vi "SPL Calc 2.0.vi"(9 "Gain":dbl(slide) min=0.0 max=50.0 scale=0.0..50.0, 10 "Voltage RMS Reference (V RMS/Pa)":dbl, 11 "Dynamic Data":dynamicdata(waveform)) -> (3 "SPL":dbl)   [LabVIEW 2020]
uses:
  <vilib>/measure/madcrms.llb/Basic Averaged DC-RMS for 1 Chan.vi
  <vilib>/measure/NI_MAPro.lvlib
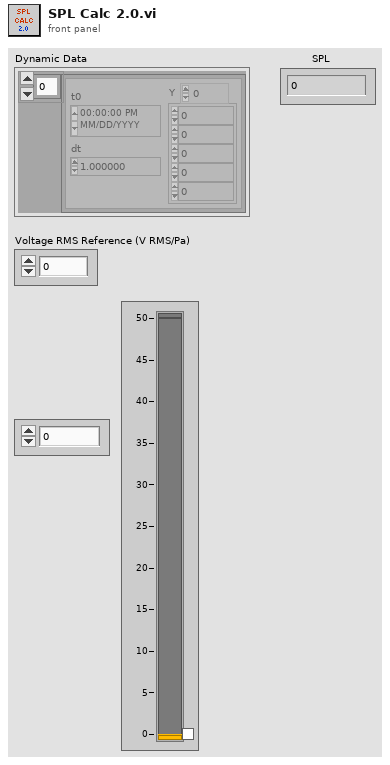
[diagram p1: front panel]
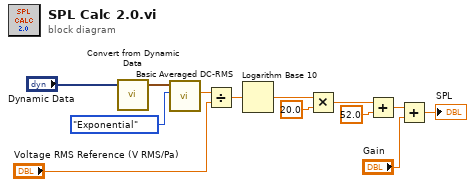
[diagram p0: block diagram]
diagram:
  n1 = call "Convert from Dynamic Data"("Dynamic Data Type"="Dynamic Data") -> ("Waveform"=w2:waveform(dbl))  [unwired: 3 in]
  n2 = call-poly <vilib>:"Basic Averaged DC-RMS.vi"("averaging type"=enum16{"Linear", "Exponential"}."Exponential", "signal in"=w2) -> ("RMS value"=w5:dbl)  [unwired: 6 in, 3 out]
  n3 = Divide(x=w5, y="Voltage RMS Reference (V RMS/Pa)") -> (x/y=w6:dbl)
  n4 = Logarithm Base 10(1:w6) -> (0:w7:dbl)
  n5 = Multiply(x=w7, y=20.0) -> (x*y=w10:dbl)
  n6 = Add(x=w10, y=52.0) -> (x+y=w11:dbl)
  n7 = Add(x=w11, y="Gain") -> (x+y=→"SPL":dbl)
